vi "Write Max Current.vi"(10 "Max Current":dbl, 11 "E3610x in":refnum<class "E3610x.lvclass">) -> (3 "E3610x out":refnum<class "E3610x.lvclass">)   [LabVIEW 2020, in "E3610x.lvclass"]
uses:
  E3610x.lvclass
  E3610x.lvclass/E3610x.ctl
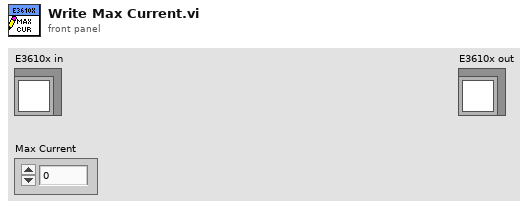
[diagram p1: front panel]
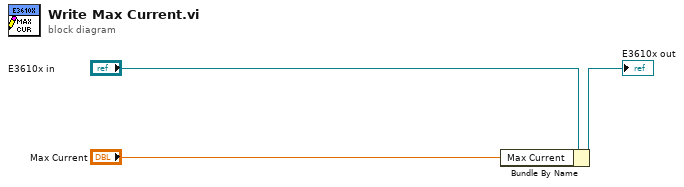
[diagram p0: block diagram]
diagram:
  n1 = Bundle By Name(cluster="E3610x in", "Max Current"="Max Current") -> (→"E3610x out":refnum<class "E3610x.lvclass">)
